vi "FTW-Example-SLASD-Core-Initialize.vi"(0 "Initialization Sequence":string, 5 "FTW Actor Instance Configuration":string, 11 "error in (no error)":errorcluster) -> (4 "Actor Template-Core out":refnum<class "FTW-Example-SLASD-Core.lvclass">, 6 "Incoming Requests":refnum<event-registration>, 15 "error out":errorcluster)   [LabVIEW 2018, in "FTW-Example-SLASD-Core.lvclass"]
uses:
  FTW-Example-SLASD-Core.lvclass
  source/CodeGen/JSON Deserialize/FTW-JSON-Deserialize.xnode
  source/actor/Publisher/FTW-Publisher.lvclass
  source/CodeGen/JSON Deserialize/FTW-JSON-Core-GetFlattenedValue.vi
  source/Reflection/FTW-Reflection-Type.vi
  source/JSON/core/FTW-JSON-Core-EncodingFlags.vi
  source/JSON/FTW-JSON-Parse.vi
  source/actor/Message/Request/FTW-Message-IncomingRequest.lvclass
  C:/Jobs/Featherweight/featherweight-2018/source/actor/Message/Base/FTW-Message.lvclass
  source/actor/Message/Base/FTW-Message.lvclass
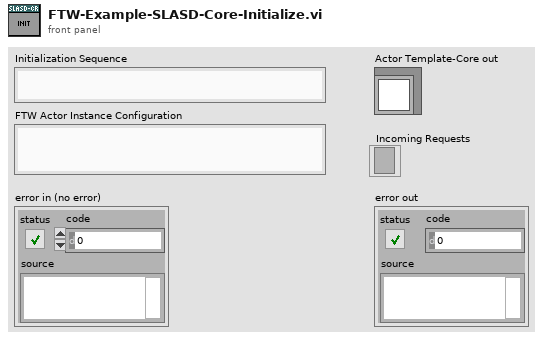
[diagram p1: front panel]
types:
  T1 = cluster{"Incoming Requests":refnum<event-registration>, "Local Messages":refnum<event-registration>, "Subscriber Registration":refnum<event-registration>}
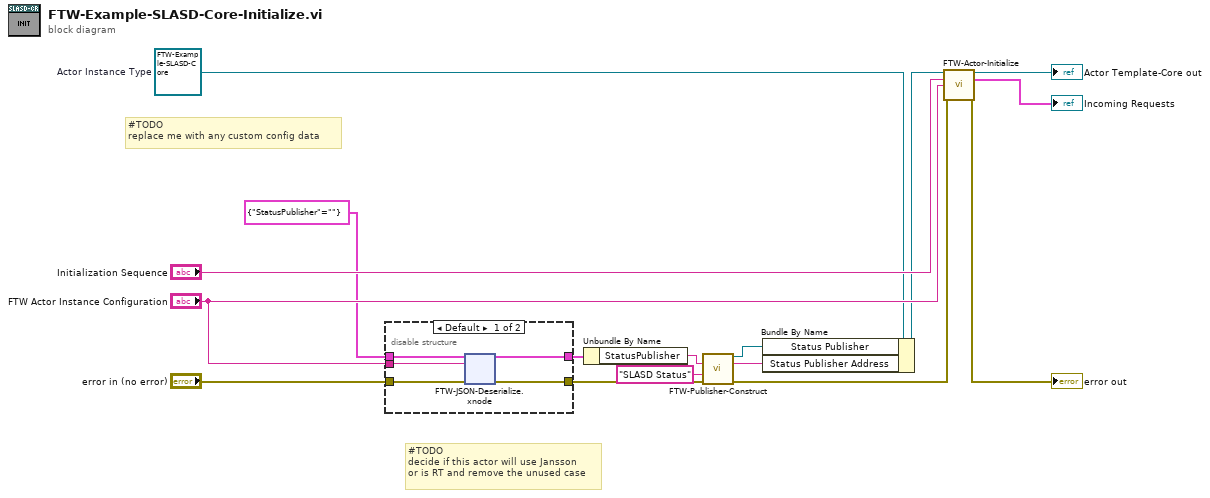
[diagram p0: block diagram]
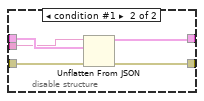
[diagram p2: hidden frame]
diagram:
  w7 = refnum<class "FTW-Example-SLASD-Core.lvclass"> refnum  # Actor Instance Type
  # "#TODO\ndecide if this actor will use Jansson\nor is RT and remove the unused case"
  # "#TODO\nreplace me with any custom config data"
  n1 = disable-structure shown="Default" {
    disable-tunnel: "error in (no error)" -> [w21 w38]
    disable-tunnel: [w20 w37] -> w11
    disable-tunnel: "FTW Actor Instance Configuration" -> [w19 w35]
    disable-tunnel: cluster{"StatusPublisher":string} {"StatusPublisher"=""} ("Type and Defaults") -> [w18 w36]
    disable-tunnel: [w17 w34] -> w8
    frame condition #0 (active) {
      n2 = xnode "FTW-JSON-Deserialize.xnode"("Type and Defaults"=w18, "JSON String"=w19, "error in"=w21) -> ("Values"=w17:cluster{"StatusPublisher":string}, "error out"=w20:errorcluster)
    }
    frame condition #1 {
      n3 = Unflatten From JSON(JSON string=w35, type and defaults=w36, error in (no error)=w38) -> (value=w34:cluster{"StatusPublisher":string}, error out=w37:errorcluster)  [unwired: 4 in]
    }
  }
  n4 = Unbundle By Name(w8) -> ("StatusPublisher"=w5:string)
  n5 = call "FTW-Publisher-Construct.vi"("Address"=w5, "Identity"="SLASD Status", "error in"=w11) -> ("FTW-Publisher Out"=w2:refnum<class "FTW-Publisher.lvclass">, "Actual Address"=w1:string, "error out"=w6:errorcluster)  [unwired: 10 in]
  n6 = Bundle By Name(cluster=w7, "Status Publisher"=w2, "Status Publisher Address"=w1) -> (w3:refnum<class "FTW-Example-SLASD-Core.lvclass">)
  n7 = call-dynamic "FTW-Actor-Initialize.vi"("FTW Actor Instance Type"=w3, "Initialization Job Sequence"="Initialization Sequence", "Actor Instance Configuration"="FTW Actor Instance Configuration", "error in"=w6) -> ("FTW Actor Instance"=→"Actor Template-Core out":refnum<class "FTW-Example-SLASD-Core.lvclass">, "Event Refnums"=→"Incoming Requests":T1, "error out"=→"error out":errorcluster)  [unwired: 9 in]
